vi "F5790 Config Panel.vi"(8 "error in (no error)":errorcluster, 11 "F5790 session in":T1) -> (0 "error out":errorcluster, 3 "F5790 session out":T1)   [LabVIEW 2020]
doc: "Config panel of ACMS Fluke 5790."
uses:
  F5790 session.ctl
panel:
  in  "btn test":bool
  in  "btn ok":bool
  in  "ext guard":bool caption="External guard"
  in  "Digital filter mode":enum16{"off", "fast", "medium", "slow"}(ring)
  in  "High resolution":enum16{"off", "on"}(ring)
  in  "Digital filter restart":enum16{"medium", "fine", "coarse"}(ring)
  in  "Input":enum16{"input 1", "input 2", "wide-band"}(ring)
  in  "VISA":refnum<visa-resource-name>
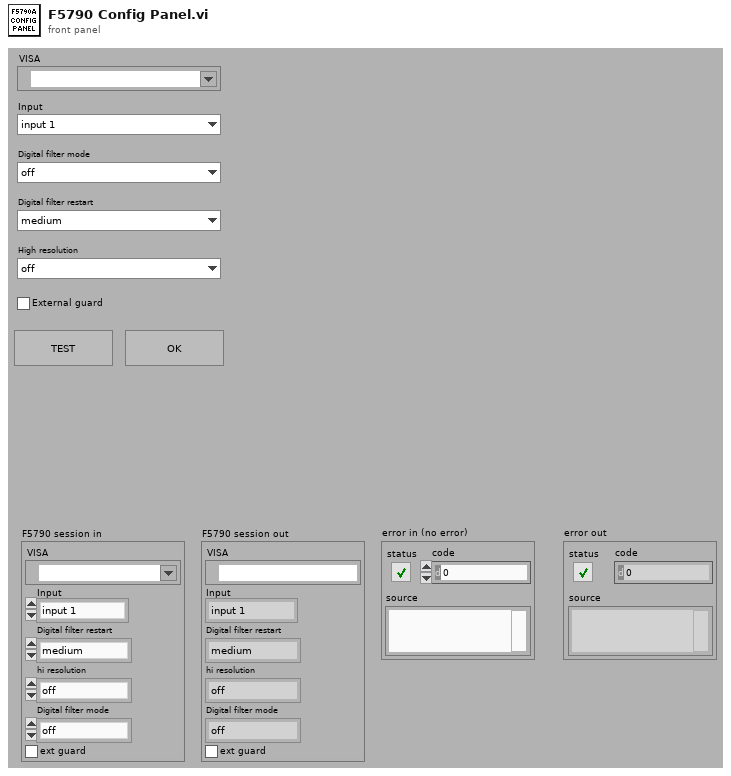
[diagram p1: front panel]
types:
  T1 = typedef "F5790 session.ctl" = cluster{"VISA":refnum<visa-resource-name>, "Input":enum16{"input 1", "input 2", "wide-band"}, "Digital filter restart":enum16{"medium", "fine", "coarse"}, "hi resolution":enum16{"off", "on"}, "Digital filter mode":enum16{"off", "fast", "medium", "slow"}, "ext guard":bool}
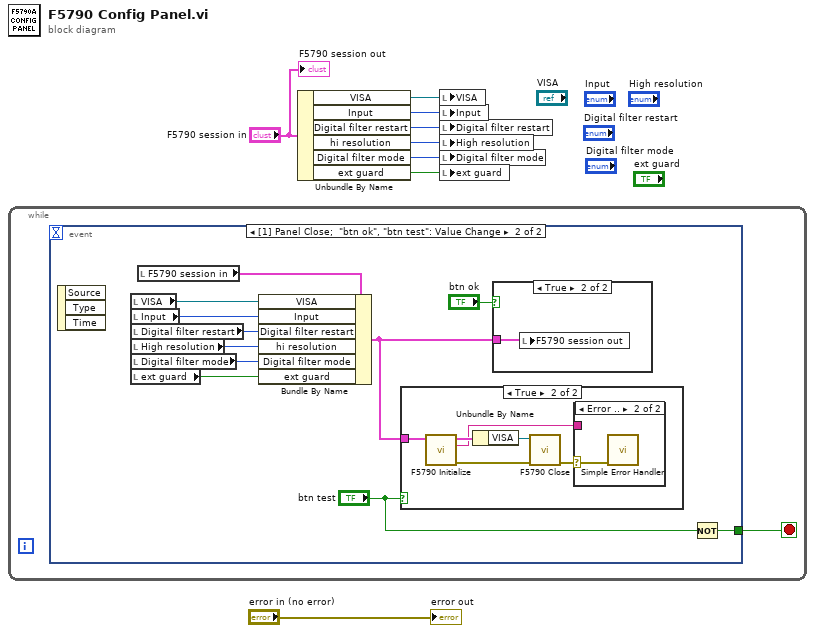
[diagram p0: block diagram]
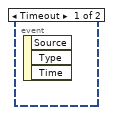
[diagram p2: hidden frame]
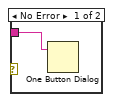
[diagram p4: hidden frame]
diagram:
  n1 = while {
    stop <- w9 stop-if-true
    n2 = event shown="[1] Panel Close;  \"btn ok\", \"btn test\": Value Change" {
      selector: _ -> [_ _]
      dyn-events: _ -> [_ _]
      timeout: _ -> [_ _]
      tunnel: [_ w11] -> w9
      event Timeout {
        n3 = event-data() -> ()  [unwired: 1 in, 3 out]
      }
      event Panel Close; "btn ok", "btn test": Value Change {
        n4 = event-data() -> ()  [unwired: 1 in, 3 out]
        n5 = local read "VISA"() -> (w20:refnum<visa-resource-name>)
        n6 = local read "Input"() -> (w19:enum16{"input 1", "input 2", "wide-band"})
        n7 = local read "Digital filter restart"() -> (w18:enum16{"medium", "fine", "coarse"})
        n8 = local read "High resolution"() -> (w17:enum16{"off", "on"})
        n9 = local read "Digital filter mode"() -> (w16:enum16{"off", "fast", "medium", "slow"})
        n10 = local read "ext guard"() -> (w15:bool)
        n11 = local read "F5790 session in"() -> (w14:T1)
        n12 = Bundle By Name(cluster=w14, "VISA"=w20, "Input"=w19, "Digital filter restart"=w18, "hi resolution"=w17, "Digital filter mode"=w16, "ext guard"=w15) -> (w10:T1)
        n13 = case shown="True" "btn test" {
          tunnel: w10 -> [_ w26]
          frame False {
          }
          frame True {
            n14 = call "F5790 Initialize.vi"("F5790 session"=w26) -> ("error out"=w25:errorcluster, "ID"=w21:string, "F5790 session out"=w24:T1)  [unwired: 8 in]
            n15 = Unbundle By Name(w24) -> ("VISA"=w23:refnum<visa-resource-name>)
            n16 = call "F5790 Close.vi"("error in (no error)"=w25, "VISA in"=w23) -> ("error out"=w22:errorcluster)  [unwired: 9 in]
            n17 = case shown="Error .." w22 {
              selector: w22 -> [_ w28]
              tunnel: w21 -> [w27 _]
              frame No Error {
                n18 = One Button Dialog(message=w27) -> ()  [unwired: 1 in, 1 out]
              }
              frame Error {
                n19 = call <vilib>:"Simple Error Handler.vi"("error in (no error)"=w28) -> ()  [unwired: 4 in, 5 out]
              }
            }
          }
        }
        n20 = case shown="True" "btn ok" {
          tunnel: w10 -> [_ w29]
          frame False {
          }
          frame True {
            n21 = local write "F5790 session out"(w29) -> ()
          }
        }
        n22 = Not(x="btn test") -> (.not. x?=w11:bool)
      }
    }
  }
  n23 = Unbundle By Name("F5790 session in") -> ("VISA"=w7:refnum<visa-resource-name>, "Input"=w6:enum16{"input 1", "input 2", "wide-band"}, "Digital filter restart"=w5:enum16{"medium", "fine", "coarse"}, "hi resolution"=w4:enum16{"off", "on"}, "Digital filter mode"=w3:enum16{"off", "fast", "medium", "slow"}, "ext guard"=w1:bool)
  n24 = local write "VISA"(w7) -> ()
  n25 = local write "Input"(w6) -> ()
  n26 = local write "Digital filter restart"(w5) -> ()
  n27 = local write "High resolution"(w4) -> ()
  n28 = local write "Digital filter mode"(w3) -> ()
  n29 = local write "ext guard"(w1) -> ()
  "F5790 session out" <- "F5790 session in"
  "error out" <- "error in (no error)"
